vi "(SubVI) Average 2D array.vi"(3 "Transpose?":bool, 4 "Array":dbl[][](array[numeric])) -> (1 "Avg. Array":dbl[](array[numeric]))   [LabVIEW 2014]
panel:
  out "size(s) 3":i32
  out "size(s) 2":i32
  out "size(s)":i32[](array[numeric])
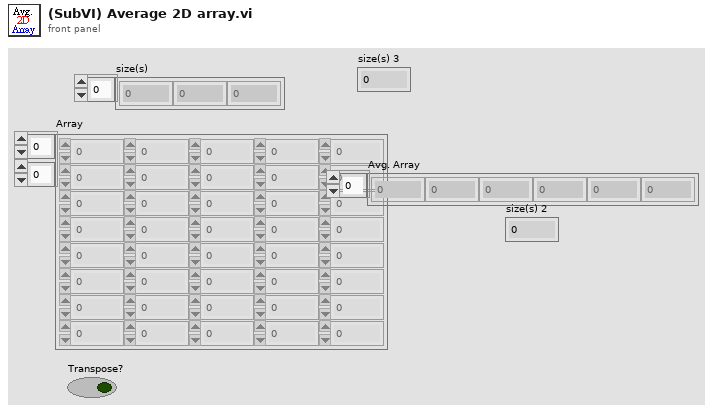
[diagram p1: front panel]
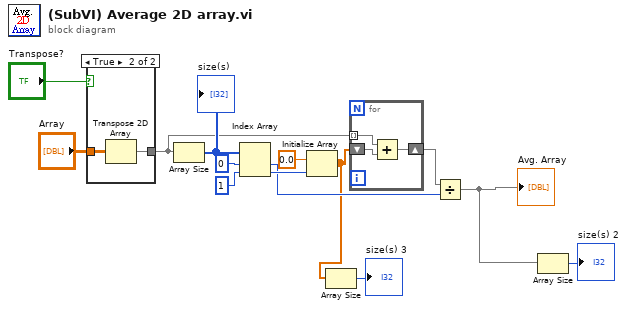
[diagram p0: block diagram]
diagram:
  n1 = case shown="True" "Transpose?" {
    tunnel: "Array" -> [w15 w17]
    tunnel: [w15 w16] -> w6
    frame False {
    }
    frame True {
      n2 = Transpose 2D Array(2D array=w17) -> (transposed array=w16:dbl[][])
    }
  }
  n3 = Array Size(array=w6) -> (size(s)=w13:i32[])
  "size(s)" <- w13
  n4 = Index Array(array=w13, index #1=0 ("index"), index #2=1 ("index")) -> (element #1=w8:i32, element #2=w10:i32)
  n5 = Initialize Array(0.0 ("element"), w10) -> (w2:dbl[])
  n6 = Array Size(array=w2) -> (size(s)=→"size(s) 3":i32)
  n7 = for {
    shift-right: [w18] -> w9
    shift-left: w2 -> [w20]
    tunnel: w6 -> [w19] mode=indexing
    n8 = Add(x=w19, y=w20) -> (x+y=w18:dbl[])
  }
  n9 = Divide(x=w9, y=w8) -> (x/y=w4:dbl[])
  "Avg. Array" <- w4
  n10 = Array Size(array=w4) -> (size(s)=→"size(s) 2":i32)
